vi "tester.vi"() -> ()   [LabVIEW 2021]
uses:
  a4a16baf-7f12-4938-921f-594048da5a8b.vi
  <vilib>/nisyscfg/Close (System).vi
  <vilib>/nisyscfg/nisyscfg.lvlib
panel:
  in  "Refresh Button":bool
  in  "Tree":string(tree)
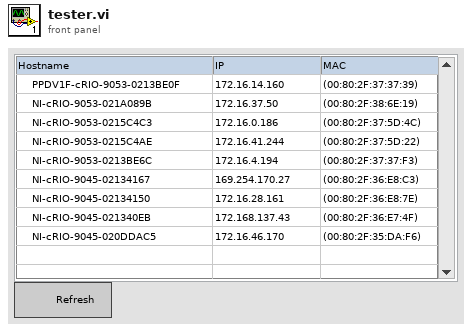
[diagram p1: front panel]
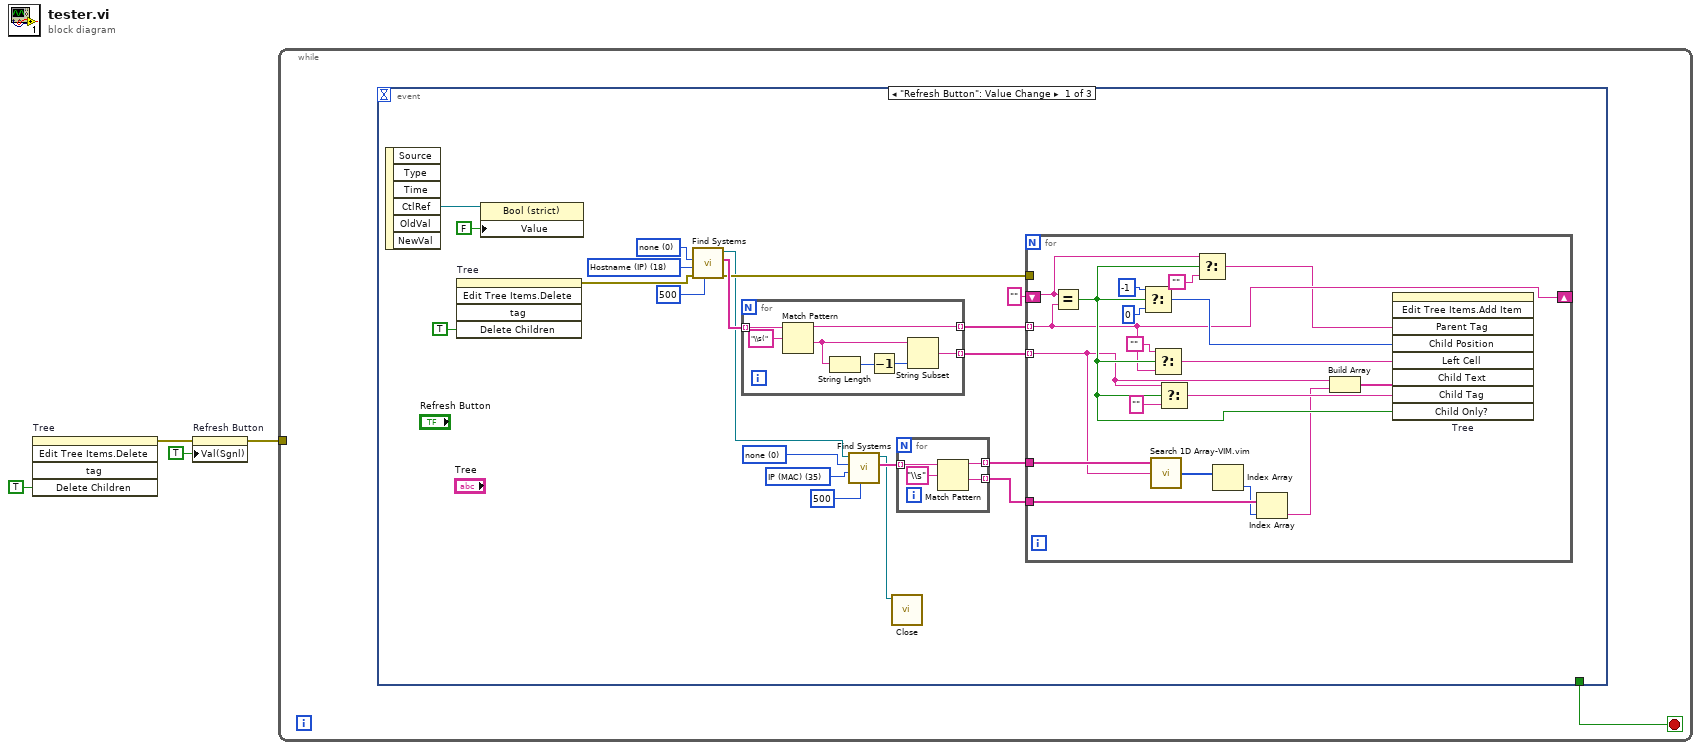
[diagram p0: block diagram]
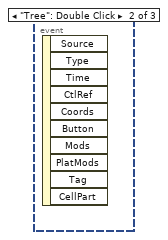
[diagram p2: hidden frame]
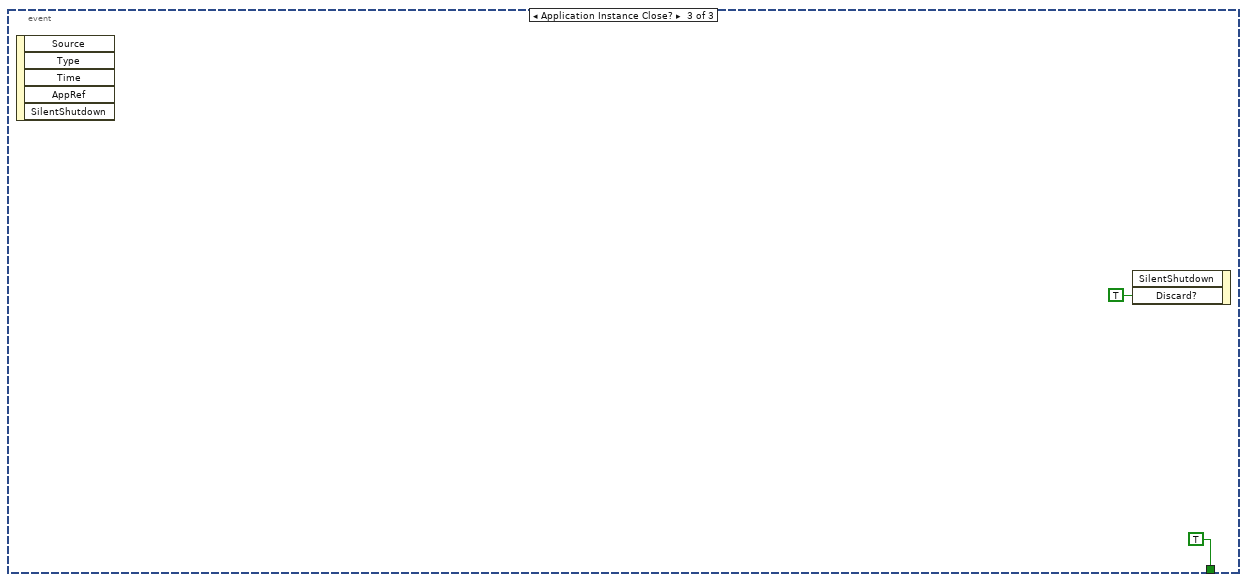
[diagram p3: hidden frame]
diagram:
  n1 = invoke on="Tree" class="Tree (strict)" method="Edit Tree Items.Delete"("Delete Children"=TRUE ("Delete Children?")) -> (error out=w3:errorcluster)  [unwired: 4 in, 4 out]
  n2 = property on="Refresh Button" class="Bool (strict)"(error in=w3, "Val(Sgnl)"=TRUE ("Value (Signaling)")) -> (error out=w2:errorcluster)  [unwired: 1 in, 1 out]
  n3 = while {
    tunnel: w2 -> [_]
    stop <- w5 stop-if-true
    n4 = event shown="[0] \"Refresh Button\": Value Change" {
      selector: _ -> [_ _ _]
      dyn-events: _ -> [_ _ _]
      timeout: _ -> [_ _ _]
      tunnel: [_ _ TRUE] -> w5
      event "Refresh Button": Value Change {
        w15 = u32 0 items=["none"=0, "only if online"=1, "all"=3] ("Include Cached Results (all)")
        w16 = u32 35 items=["Hostname"=16, "Hostname (IP)"=18, "Hostname (MAC)"=19, "IP"=32, "IP (Hostname)"=33, "IP (MAC)"=35, "MAC"=48, "MAC (Hostname)"=49, "MAC (IP)"=50] ("Output (Hostname and IP)")
        w11 = u32 0 items=["none"=0, "only if online"=1, "all"=3] ("Include Cached Results (all)")
        w12 = u32 18 items=["Hostname"=16, "Hostname (IP)"=18, "Hostname (MAC)"=19, "IP"=32, "IP (Hostname)"=33, "IP (MAC)"=35, "MAC"=48, "MAC (Hostname)"=49, "MAC (IP)"=50] ("Output (Hostname and IP)")
        n5 = event-data() -> ("CtlRef"=w7:refnum<vi>)  [unwired: 1 in, 5 out]
        n6 = invoke on="Tree" class="Tree (strict)" method="Edit Tree Items.Delete"("Delete Children"=TRUE ("Delete Children?")) -> (error out=w20:errorcluster)  [unwired: 4 in, 4 out]
        n7 = property class="Bool (strict)"(reference=w7, "Value"=FALSE) -> ()  [unwired: 1 in, 2 out]
        n8 = call <vilib>:"Find Systems.vi"("Timeout (4000 ms)"=u32 500, "error in (no error)"=w20, "Output (Hostname and IP)"=w12, "Include Cached Results (all)"=w11) -> ("error out"=w18:errorcluster, "Detected Systems"=w19:string[], "Session out"=w9:refnum<k21>)  [unwired: 5 in]
        n9 = for {
          tunnel: w19 -> [w36] mode=indexing
          tunnel: [w34] -> w21 mode=indexing
          tunnel: [w32] -> w22 mode=indexing
          n10 = Match Pattern(string=w36, regular expression="\\s(") -> (before substring=w34:string, after substring=w33:string)  [unwired: 1 in, 2 out]
          n11 = String Length(string=w33) -> (length=w31:i32)
          n12 = Decrement(x=w31) -> (x-1=w30:i32)
          n13 = String Subset(string=w33, length (rest)=w30) -> (substring=w32:string)  [unwired: 1 in]
        }
        n14 = call <vilib>:"Find Systems.vi"("Timeout (4000 ms)"=u32 500, "Output (Hostname and IP)"=w16, "Include Cached Results (all)"=w15, "Session in (localhost)"=w9) -> ("Detected Systems"=w23:string[], "Session out"=w8:refnum<k21>)  [unwired: 5 in, 1 out]
        n15 = call-poly <vilib>:"Close.vi"("Session in"=w8) -> ()  [unwired: 10 in, 1 out]
        n16 = for {
          tunnel: w23 -> [w28] mode=indexing
          tunnel: [w27] -> w24 mode=indexing
          tunnel: [w26] -> w25 mode=indexing
          n17 = Match Pattern(string=w28, regular expression="\\s") -> (before substring=w27:string, after substring=w26:string)  [unwired: 1 in, 2 out]
        }
        n18 = for {
          tunnel: w18 -> [_]
          tunnel: w21 -> [w45] mode=indexing
          tunnel: w22 -> [w38] mode=indexing
          shift-right: [w45] -> _
          shift-left: "" ("String") -> [w49]
          tunnel: w24 -> [w43]
          tunnel: w25 -> [w41]
          n19 = Equal?(x=w49, y=w45) -> (x = y?=w47:bool)
          n20 = Select(t=-1, s=w47, f=0 ("Child Position")) -> (s? t:f=w53:i32)
          n21 = call "Search 1D Array-VIM.vim"("Array"=w43, "Search Element(s)"=w38) -> ("Indices of Elements"=w42:i32[])  [unwired: 7 in]
          n22 = Select(t="", s=w47, f=w45) -> (s? t:f=w46:string)
          n23 = Select(t=w38, s=w47, f="") -> (s? t:f=w51:string)
          n24 = Select(t=w49, s=w47, f="") -> (s? t:f=w37:string)
          n25 = Index Array(array=w42) -> (element=w40:i32)  [unwired: 1 in]
          n26 = Index Array(array=w41, index=w40) -> (element=w39:string)
          n27 = Build Array(w38, w39) -> (w50:string[])
          n28 = invoke on="Tree" class="Tree (strict)" method="Edit Tree Items.Add Item"("Parent Tag"=w37, "Child Position"=w53, "Left Cell"=w46, "Child Text"=w50, "Child Tag"=w51, "Child Only?"=w47) -> ()  [unwired: 3 in, 9 out]
        }
      }
      event "Tree": Double Click {
        n29 = event-data() -> ()  [unwired: 1 in, 10 out]
      }
      event Application Instance Close? {
        n30 = event-data() -> ()  [unwired: 1 in, 5 out]
        n31 = event-data("Discard?"=TRUE) -> ()  [unwired: 2 in, 1 out]
      }
    }
  }
